vi "LSCI332 GetRelayOutput.vi"(0 "VISA Rsrc":refnum<visa-resource-name>="GPIB0::12::INSTR", 5 "Relay(1)":u32(ring) caption="Relay" items=["Relay 1", "Relay 2"], 11 "error in":errorcluster) -> (4 "RelayMode":enum16{"Off", "On", "Alarm"}(ring) caption="Relay Mode", 6 "Alarm Input":enum16{"A", "B"}(ring), 8 "Alarm Type":enum16{"Low", "High", "Low&High"}(ring), 15 "error out":errorcluster)   [LabVIEW 2019]
doc: "Ce Vi nterroge l'instrument sur la valeur de \"Manual output\" de chauffage actuelle, en %."
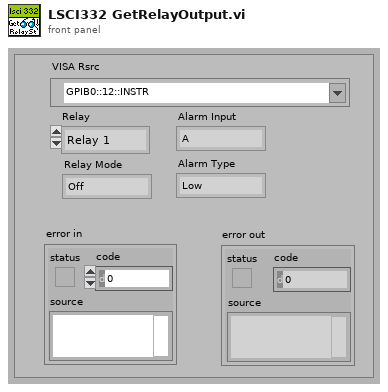
[diagram p1: front panel]
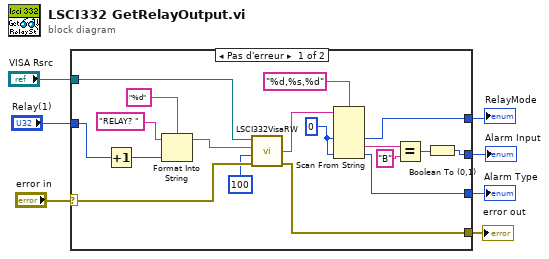
[diagram p0: block diagram]
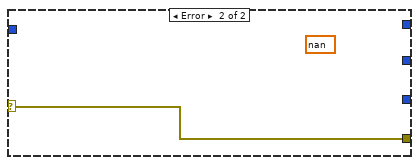
[diagram p2: hidden frame]
diagram:
  n1 = case shown="Pas d'erreur" "error in" {
    selector: "error in" -> [w24 w26]
    tunnel: [w22 w26] -> w7
    tunnel: "VISA Rsrc" -> [w25 _]
    tunnel: "Relay(1)" -> [w21 _]
    tunnel: [w14 _] -> w3
    tunnel: [w9 _] -> w2
    tunnel: [w8 _] -> w1
    frame No Error {
      w13 = u16 0 ("Nbcaract")
      n2 = Increment(x=w21) -> (x+1=w15:u32)
      n3 = Format Into String(format string="%d", initial string="RELAY? ", w15) -> (resulting string=w19:string)  [unwired: 1 in, 1 out]
      n4 = call <userlib>:"LSCI332VisaRW.vi"("error in (no error)"=w24, "Nbcaract"=u32 100, "ChaineCom"=w19, "VISA Rsrc"=w25) -> ("error out"=w22:errorcluster, "ChaineRep"=w18:string)  [unwired: 3 in, 2 out]
      n5 = Scan From String(format string="%d,%s,%d", input string=w18, default 1=w13, default 3=w13) -> (output 1=w14:u16, output 2=w12:string, output 3=w8:u16)  [unwired: 3 in, 3 out]
      n6 = Equal?(x=w12, y="B") -> (x = y?=w10:bool)
      n7 = Boolean To (0,1)(Boolean=w10) -> (0, 1=w9:i16)
    }
    frame Error {
      (unwired) nan ("default value 1")
    }
  }
  "error out" <- w7
  "RelayMode" <- w3
  "Alarm Type" <- w1
  "Alarm Input" <- w2
